vi "Register Graph.vi"(8 "error in (no error)":errorcluster, 10 "Graph Reference":refnum<vi>, 11 "Graph Manager in":refnum<class "Graph Manager.lvclass">) -> (0 "error out":errorcluster, 3 "Graph Manager out":refnum<class "Graph Manager.lvclass">)   [LabVIEW 2016, in "Graph Manager.lvclass"]
uses:
  Graph Manager.lvclass
  Graph Manager.lvclass/Graph Manager.ctl
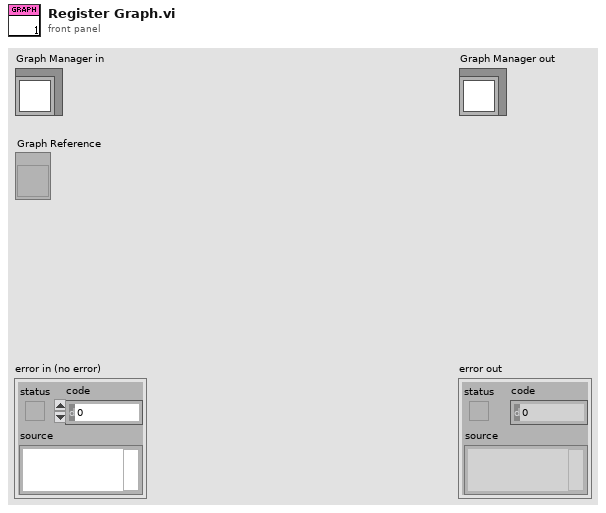
[diagram p1: front panel]
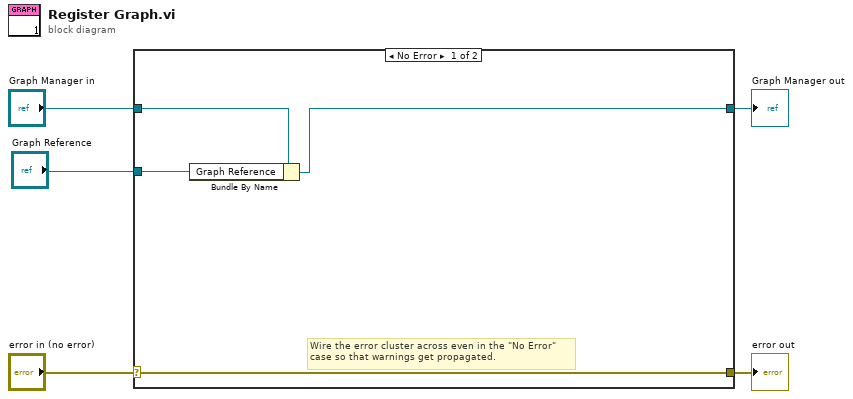
[diagram p0: block diagram]
diagram:
  n1 = case shown="No Error" "error in (no error)" {
    selector: "error in (no error)" -> [w9 w11]
    tunnel: [w9 w11] -> w4
    tunnel: [w6 w10] -> w2
    tunnel: "Graph Manager in" -> [w8 w10]
    tunnel: "Graph Reference" -> [w7 _]
    frame No Error {
      # "Wire the error cluster across even in the \"No Error\"\ncase so that warnings get propagated."
      n2 = Bundle By Name(cluster=w8, "Graph Reference"=w7) -> (w6:refnum<class "Graph Manager.lvclass">)
    }
    frame Error {
    }
  }
  "error out" <- w4
  "Graph Manager out" <- w2
